vi "FIR e IIR.vi"() -> ()   [LabVIEW 2018]
uses:
  <vilib>/measure/macond.llb/FIR Filter for 1 Chan.vi
  <vilib>/measure/maspectr.llb/FFT Spectrum (Mag-Phase) for 1 Chan.vi
  <vilib>/measure/macond.llb/IIR Filter for 1 Chan.vi
  <vilib>/measure/NI_MABase.lvlib
  <vilib>/measure/NI_MAPro.lvlib
panel:
  out "Spectrum 2":cluster{"f0":dbl, "df":dbl, "magnitude":dbl[]}(graph)
  out "Signal 2":waveform(dbl)[](graph) caption="Signal"
  in  "optional IIR filter specifications":T1={"Lower PB"=100.0, "Upper PB"=0.0, "Lower SB"=200.0, "Upper SB"=0.0, "PB Gain"=-3.0, "SB Gain"=-60.0, "Scale"=TRUE} {"PB Gain" format="%0.2f"; "SB Gain" format="%0.2f"; "Lower SB" format="%0.2p"; "Upper SB" format="%0.2f"; "Lower PB" format="%0.2p"; "Upper PB" format="%0.2f"}
  in  "IIR filter specifications":T2={"Topology"=enum."Butterworth", "Type"=enum."Lowpass", "Order"=1, "Lower Fc"=100.0, "Upper Fc"=200.0, "PB Ripple"=1.0, "SB Attenuation"=60.0} {"PB Ripple" format="%0.2f"; "SB Attenuation" format="%0.2f"; "Lower Fc" format="%0.2p"; "Upper Fc" format="%0.2p"}
  in  "db ON":bool
  in  "optional FIR filter specifications":T3={"PB Gain"=-3.0, "SB Gain"=-60.0, "Scale"=TRUE, "Window"=enum."Flat Top"} {"SB Gain" format="%.2p"; "PB Gain" format="%.2p"}
  in  "FIR filter specifications":T4={"Topology"=enum."Off", "Type"=enum."Lowpass", "#Taps"=50, "Lower PB"=100.0, "Upper PB"=0.0, "Lower SB"=200.0, "Upper SB"=0.0} {"Lower SB" format="%0.2p"; "Upper SB" format="%0.2p"; "Lower PB" format="%0.2p"; "Upper PB" format="%0.2p"}
  in  "Noise":dbl
  in  "Freq2":dbl(slide) scale=0.0..100.0
  in  "Freq1":dbl(slide) scale=0.0..100.0
  out "Spectrum":cluster{"f0":dbl, "df":dbl, "magnitude":dbl[]}(graph)
  out "Signal":waveform(dbl)[](graph)
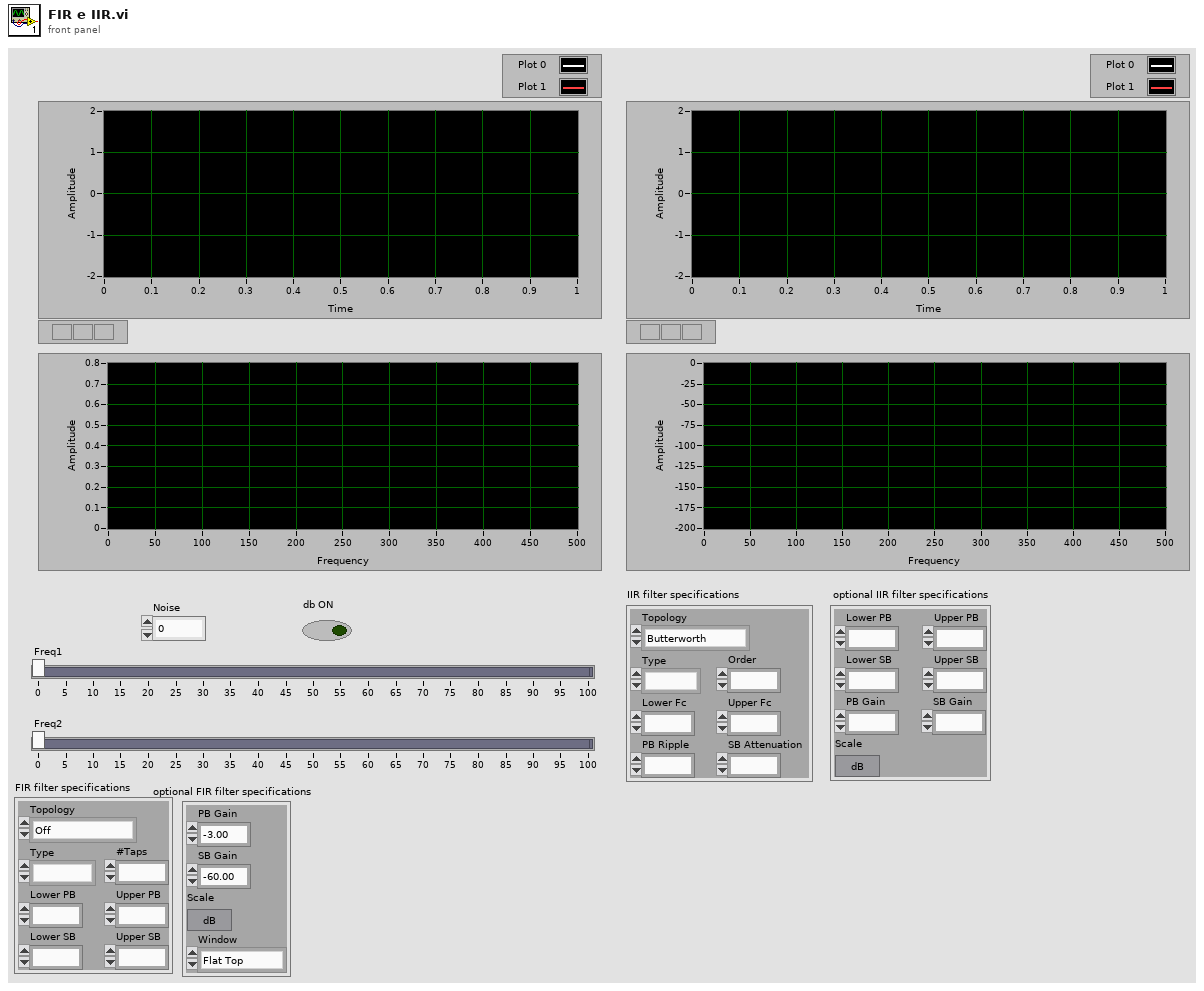
[diagram p1: front panel]
types:
  T1 = cluster{"Lower PB":dbl, "Upper PB":dbl, "Lower SB":dbl, "Upper SB":dbl, "PB Gain":dbl, "SB Gain":dbl, "Scale":bool}
  T2 = cluster{"Topology":enum16{"Off", "Butterworth", "Chebyshev", "Inverse Chebyshev", "Elliptic", "Bessel"}, "Type":enum16{"Lowpass", "Highpass", "Bandpass", "Bandstop"}, "Order":i32, "Lower Fc":dbl, "Upper Fc":dbl, "PB Ripple":dbl, "SB Attenuation":dbl}
  T3 = cluster{"PB Gain":dbl, "SB Gain":dbl, "Scale":bool, "Window":enum16{"None", "Hanning", "Hamming", "Triangular", "Blackman", "Exact Blackman", "Blackman-Harris", "Kaiser-Bessel", "Flat Top"}}
  T4 = cluster{"Topology":enum16{"Off", "FIR by Specification", "Equi-ripple FIR", "Windowed FIR"}, "Type":enum16{"Lowpass", "Highpass", "Bandpass", "Bandstop"}, "#Taps":i32, "Lower PB":dbl, "Upper PB":dbl, "Lower SB":dbl, "Upper SB":dbl}
  T5 = cluster{"dB On (F)":bool, "unwrap phase (F)":bool, "convert to degree (F)":bool}
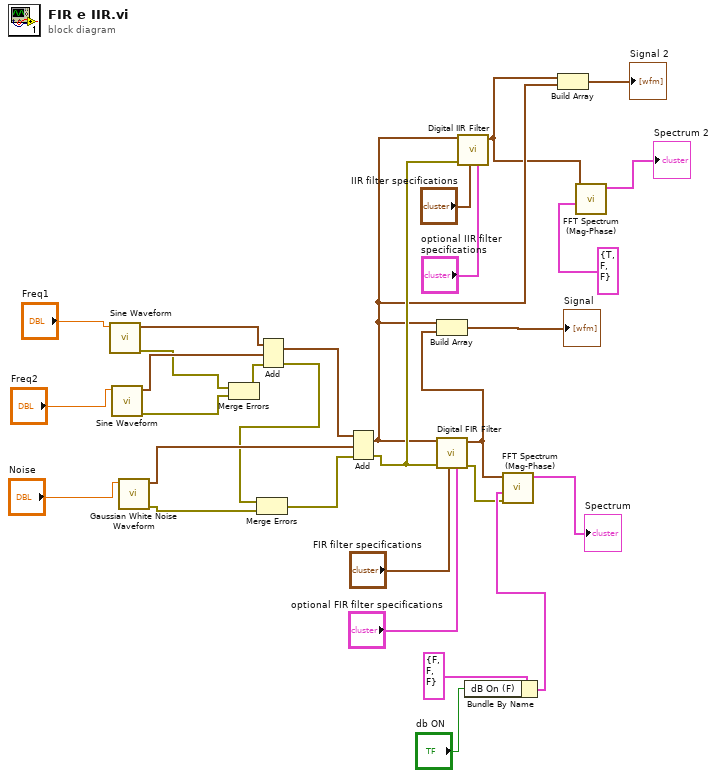
[diagram p0: block diagram]
diagram:
  n1 = call <vilib>:"Sine Waveform.vi"("frequency"="Freq1") -> ("error out"=w23:errorcluster, "signal out"=w27:waveform(dbl))  [unwired: 9 in]
  n2 = call <vilib>:"Sine Waveform.vi"("frequency"="Freq2") -> ("error out"=w24:errorcluster, "signal out"=w26:waveform(dbl))  [unwired: 9 in]
  n3 = call <vilib>:"Gaussian White Noise Waveform.vi"("standard deviation"="Noise") -> ("error out"=w18:errorcluster, "signal out"=w21:waveform(dbl))  [unwired: 9 in]
  n4 = Merge Errors(w23, w24) -> (w25:errorcluster)
  n5 = Add(1:w26, 2:w27, 4:w25) -> (0:w22:waveform(dbl), 3:w19:errorcluster)
  n6 = Merge Errors(w19, w18) -> (w20:errorcluster)
  n7 = Add(1:w21, 2:w22, 4:w20) -> (0:w4:waveform(dbl), 3:w9:errorcluster)
  n8 = call-poly <vilib>:"Digital FIR Filter.vi"("optional FIR filter specifications"="optional FIR filter specifications", "FIR filter specifications"="FIR filter specifications", "error in (no error)"=w9, "signal in"=w4) -> ("error out"=w8:errorcluster, "signal out"=w13:waveform(dbl))  [unwired: 5 in, 1 out]
  n9 = Build Array(w4, w13) -> (→"Signal":waveform(dbl)[])
  n10 = call-poly <vilib>:"Digital IIR Filter.vi"("optional IIR filter specifications"="optional IIR filter specifications", "IIR filter specifications"="IIR filter specifications", "error in (no error)"=w9, "signal in"=w4) -> ("signal out"=w3:waveform(dbl))  [unwired: 5 in, 2 out]
  n11 = Bundle By Name "Bundle By Name"(cluster=T5 {"dB On (F)"=FALSE, "unwrap phase (F)"=FALSE, "convert to degree (F)"=FALSE} ("view"), "dB On (F)"="db ON") -> (w11:T5)
  n12 = call-poly <vilib>:"FFT Spectrum (Mag-Phase).vi"("error in (no error)"=w8, "view"=w11, "time signal"=w13) -> ("magnitude"=→"Spectrum":cluster{"f0":dbl, "df":dbl, "magnitude":dbl[]})  [unwired: 4 in, 4 out]
  n13 = Build Array(w3, w4) -> (→"Signal 2":waveform(dbl)[])
  n14 = call-poly <vilib>:"FFT Spectrum (Mag-Phase).vi"("view"=T5 {"dB On (F)"=TRUE, "unwrap phase (F)"=FALSE, "convert to degree (F)"=FALSE}, "time signal"=w3) -> ("magnitude"=→"Spectrum 2":cluster{"f0":dbl, "df":dbl, "magnitude":dbl[]})  [unwired: 5 in, 4 out]
